vi "timesignatures.vi"(11 "Time Signatures":T1) -> (3 "appended array":i32[][](array[numeric]))   [LabVIEW 2019]
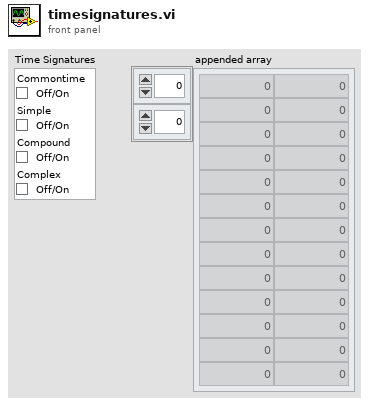
[diagram p1: front panel]
types:
  T1 = cluster{"Commontime":bool, "Simple":bool, "Compound":bool, "Complex":bool}
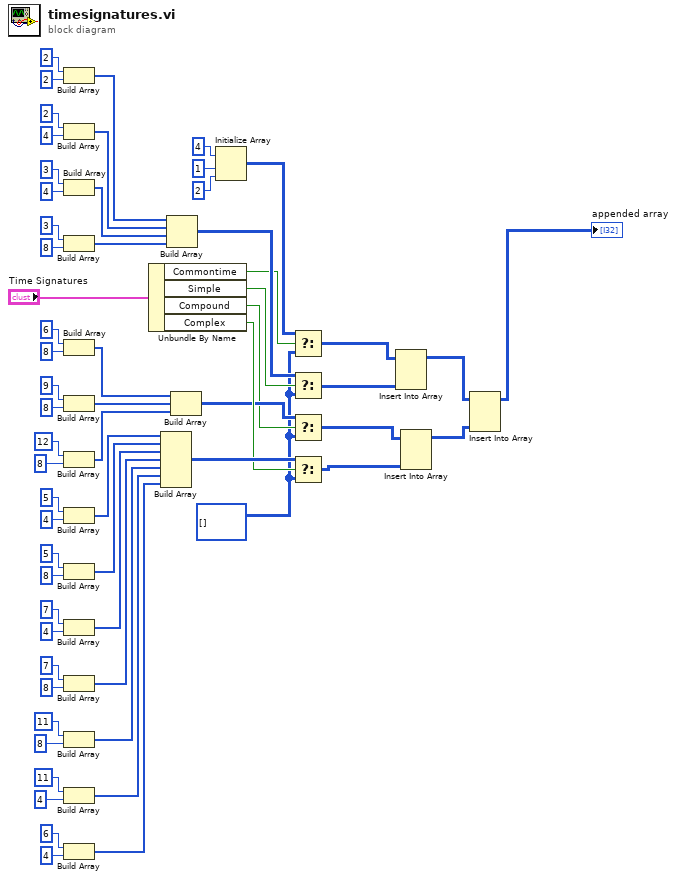
[diagram p0: block diagram]
diagram:
  w8 = i32[][] [] ("appended array")
  n1 = Build Array(2, 2) -> (w23:i32[])
  n2 = Build Array(2, 4) -> (w24:i32[])
  n3 = Build Array(3, 4) -> (w25:i32[])
  n4 = Build Array(3, 8) -> (w26:i32[])
  n5 = Build Array(6, 8) -> (w35:i32[])
  n6 = Build Array(9, 8) -> (w36:i32[])
  n7 = Build Array(12, 8) -> (w37:i32[])
  n8 = Build Array(5, 4) -> (w54:i32[])
  n9 = Build Array(5, 8) -> (w55:i32[])
  n10 = Build Array(7, 4) -> (w56:i32[])
  n11 = Build Array(7, 8) -> (w57:i32[])
  n12 = Build Array(11, 8) -> (w58:i32[])
  n13 = Build Array(11, 4) -> (w59:i32[])
  n14 = Build Array(6, 4) -> (w60:i32[])
  n15 = Unbundle By Name("Time Signatures") -> ("Commontime"=w22:bool, "Simple"=w27:bool, "Compound"=w38:bool, "Complex"=w61:bool)
  n16 = Build Array(w54, w55, w56, w57, w58, w59, w60) -> (w62:i32[][])
  n17 = Build Array(w23, w24, w25, w26) -> (w28:i32[][])
  n18 = Build Array(w35, w36, w37) -> (w39:i32[][])
  n19 = Initialize Array(4 ("element"), 1 ("dimension size"), 2 ("dimension size")) -> (w9:i32[][])
  n20 = Select(t=w9, s=w22, f=w8) -> (s? t:f=w7:i32[][])
  n21 = Select(t=w28, s=w27, f=w8) -> (s? t:f=w6:i32[][])
  n22 = Select(t=w39, s=w38, f=w8) -> (s? t:f=w5:i32[][])
  n23 = Select(t=w62, s=w61, f=w8) -> (s? t:f=w4:i32[][])
  n24 = Insert Into Array(array=w7, new element=w6) -> (w3:i32[][])  [unwired: 2 in]
  n25 = Insert Into Array(array=w5, new element=w4) -> (w2:i32[][])  [unwired: 2 in]
  n26 = Insert Into Array(array=w3, new element=w2) -> (→"appended array":i32[][])  [unwired: 2 in]
